vi "全局 用户名.vi"() -> ()   [LabVIEW 2014]
panel:
  in  "用户名":string
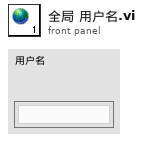
[diagram p1: front panel]
diagram:
